vi "MultisitePinMapARegistered_SessionManagementApiRoundTrip_AllNodesSucceed.vi"() -> (6 "pass":bool, 8 "result":string, 15 "error out":errorcluster)   [LabVIEW 2020]
uses:
  Pin Map Client_lv/Pin Map Client_v1/RPC Messages/ni_measurementlink_pinmap_v1_CreatePinMapFromXmlRequest.ctl
  31aaf20a-e7c9-45c8-9685-a1adea383544.vi
  030eba9d-dfb1-4c70-a755-4ca582c4358b.vi
  <vilib>/Comparison/Less/Less Functor/Less Functor.lvclass
  Session Management Client_lv/Session Management Client_v1/Session Management Client_v1.lvlib
  Pin Map Client_lv/Pin Map Client_v1/Pin Map Client_v1.lvlib
panel:
  # "Test assumes discovery service, pin map service, and session management service have already been started."
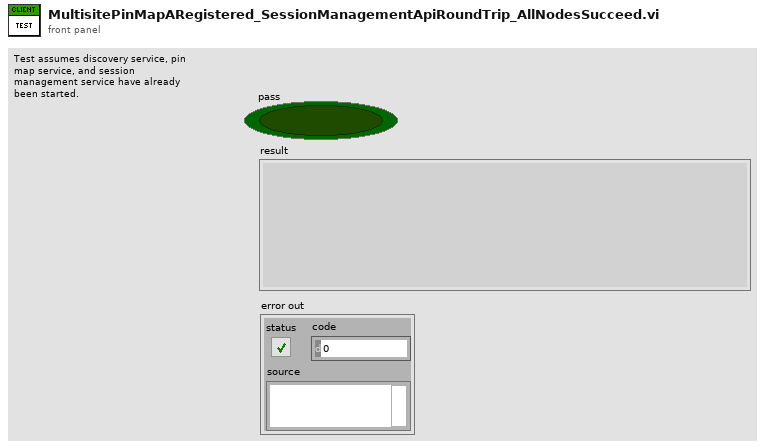
[diagram p1: front panel]
types:
  T1 = typedef "Pin Map Client_v1.lvlib/ni_measurementlink_pinmap_v1_CreatePinMapFromXmlRequest.ctl" = cluster{"pin_map_id":string, "pin_map_xml":string}
  T2 = typedef "grpc-lvsupport-release.lvlib/grpcId.ctl" = u64
  T3 = typedef "Session Management Client_v1.lvlib/ni_measurementlink_sessionmanagement_v1_ReserveSessionsRequest.ctl" = cluster{"pin_map_context":T4, "pin_or_relay_names":string[], "instrument_type_id":string, "timeout_in_milliseconds":i32}
  T4 = typedef "Session Management Client_v1.lvlib/ni_measurementlink_PinMapContext.ctl" = cluster{"pin_map_id":string, "sites":i32[]}
  T5 = cluster{"Registration Request Data":T3, "Expected instrument_type_id/session(s)":string[]}[]
  T6 = typedef "Session Management Client_v1.lvlib/ni_measurementlink_sessionmanagement_v1_ReserveSessionsResponse.ctl" = cluster{"sessions":T7[]}
  T7 = typedef "Session Management Client_v1.lvlib/ni_measurementlink_sessionmanagement_v1_SessionInformation.ctl" = cluster{"session":T8, "resource_name":string, "channel_list":string, "instrument_type_id":string, "session_exists":bool}
  T8 = typedef "Session Management Client_v1.lvlib/ni_measurementlink_sessionmanagement_v1_Session.ctl" = cluster{"name":string}
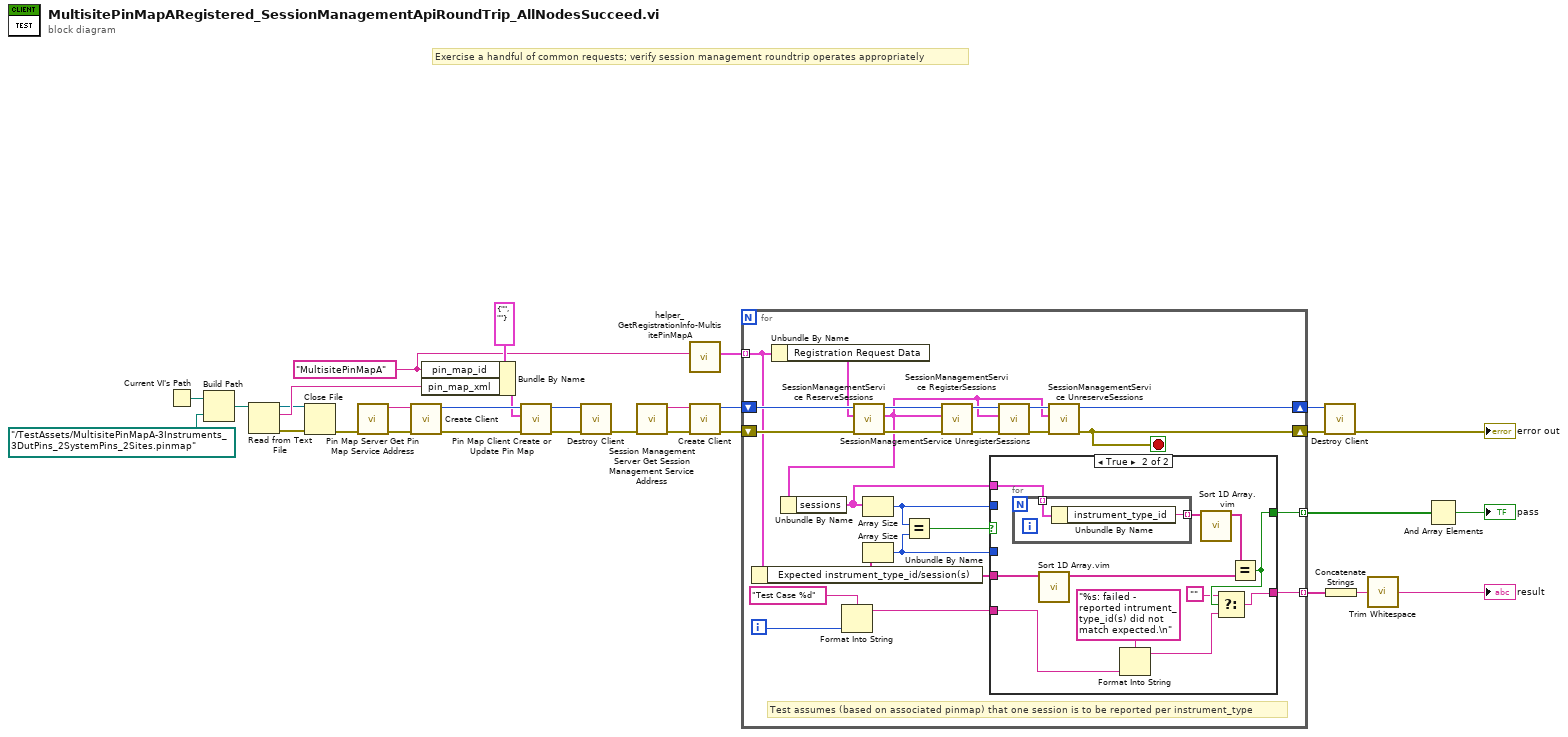
[diagram p0: block diagram]
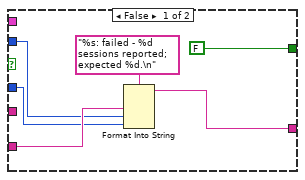
[diagram p2: hidden frame]
diagram:
  w7 = "MultisitePinMapA" ("pin_map_id")
  # "Exercise a handful of common requests; verify session management roundtrip operates appropriately"
  n1 = Current VI's Path() -> (path=w24:path)
  n2 = Build Path(base path=w24, name or relative path=path "../TestAssets/MultisitePinMapA-3Instruments_3DutPins_2SystemPins_2Sites.pinmap") -> (appended path=w22:path)
  n3 = Read from Text File(file (use dialog)=w22) -> (refnum out=w18:refnum<file>, text=w20:string, error out=w19:errorcluster)  [unwired: 3 in, 1 out]
  n4 = Close File(refnum=w18, error in=w19) -> (error out=w15:errorcluster)  [unwired: 1 out]
  n5 = call "Pin Map Server Get Pin Map Service Address.vi"("error in (no error)"=w15) -> ("error out"=w16:errorcluster, "address"=w17:string)  [unwired: 9 in]
  n6 = call "Create Client.vi"("error in"=w16, "address"=w17) -> ("error out"=w25:errorcluster, "gRPC ID Out"=w14:T2)  [unwired: 8 in]
  n7 = Bundle By Name(cluster=T1 {"pin_map_id"="", "pin_map_xml"=""} ("Request Data"), "pin_map_id"=w7, "pin_map_xml"=w20) -> (w13:T1)
  n8 = call "Pin Map Client Create or Update Pin Map.vi"("error in (no error)"=w25, "Request Data"=w13, "gRPC ID Out"=w14) -> ("error out"=w12:errorcluster, "gRPC ID out"=w11:T2)  [unwired: 6 in, 1 out]
  n9 = call "Destroy Client.vi"("error in"=w12, "gRPC ID"=w11) -> ("error out"=w10:errorcluster)  [unwired: 9 in]
  n10 = call "Session Management Server Get Session Management Service Address.vi"("error in (no error)"=w10) -> ("error out"=w29:errorcluster, "address"=w28:string)  [unwired: 9 in]
  n11 = call "helper_GetRegistrationInfo-MultisitePinMapA.vi"("Pin Map ID"=w7) -> ("Registration Request Info"=w6:T5)  [unwired: 10 in]
  n12 = call "Create Client.vi"("error in"=w29, "address"=w28) -> ("error out"=w27:errorcluster, "gRPC ID Out"=w26:T2)  [unwired: 8 in]
  n13 = for {
    shift-right: [w44] -> w8
    shift-left: w27 -> [w53]
    shift-right: [w46] -> w9
    shift-left: w26 -> [w52]
    tunnel: w6 -> [w36] mode=indexing
    tunnel: [w41] -> w5 mode=indexing
    tunnel: [w37] -> w3 mode=indexing
    i -> [w39]
    stop <- w44 stop-if-true
    # "Test assumes (based on associated pinmap) that one session is to be reported per instrument_type"
    n14 = Unbundle By Name(w36) -> ("Expected instrument_type_id/session(s)"=w31:string[])
    n15 = Unbundle By Name(w36) -> ("Registration Request Data"=w43:T3)
    n16 = Format Into String(format string="Test Case %d", w39) -> (resulting string=w38:string)  [unwired: 2 in, 1 out]
    n17 = call "SessionManagementService ReserveSessions.vi"("error in"=w53, "Request Data"=w43, "gRPC ID"=w52) -> ("error out"=w48:errorcluster, "Response Data"=w42:T6, "gRPC ID out"=w49:T2)  [unwired: 6 in]
    n18 = Unbundle By Name(w42) -> ("sessions"=w35:T7[])
    n19 = Array Size(array=w35) -> (size(s)=w33:i32)
    n20 = Array Size(array=w31) -> (size(s)=w32:i32)
    n21 = Equal?(x=w33, y=w32) -> (x = y?=w34:bool)
    n22 = call "SessionManagementService RegisterSessions.vi"("error in"=w48, "Request Data"=w42, "gRPC ID"=w49) -> ("error out"=w50:errorcluster, "gRPC ID out"=w51:T2)  [unwired: 6 in, 1 out]
    n23 = case shown="True" w34 {
      tunnel: [FALSE ("pass") w64] -> w41
      tunnel: w38 -> [w57 w60]
      tunnel: [w56 w65] -> w37
      tunnel: w35 -> [_ w70]
      tunnel: w33 -> [w55 _]
      tunnel: w32 -> [w54 _]
      tunnel: w31 -> [_ w68]
      frame False {
        n24 = Format Into String(format string="%s: failed - %d sessions reported; expected %d.\n", w57, w55, w54) -> (resulting string=w56:string)  [unwired: 2 in, 1 out]
      }
      frame True {
        n25 = for {
          tunnel: w70 -> [w72] mode=indexing
          tunnel: [w71] -> w69 mode=indexing
          n26 = Unbundle By Name(w72) -> ("instrument_type_id"=w71:string)
        }
        n27 = call "Sort 1D Array.vim"("unsorted array"=w68) -> ("sorted array"=w67:string[])  [unwired: 10 in]
        n28 = Format Into String(format string="%s: failed - reported intrument_type_id(s) did not match expected.\n", w60) -> (resulting string=w62:string)  [unwired: 2 in, 1 out]
        n29 = call "Sort 1D Array.vim"("unsorted array"=w69) -> ("sorted array"=w66:string[])  [unwired: 10 in]
        n30 = Equal?(x=w66, y=w67) -> (x = y?=w64:bool)
        n31 = Select(t="", s=w64, f=w62) -> (s? t:f=w65:string)
      }
    }
    n32 = call "SessionManagementService UnregisterSessions.vi"("error in"=w50, "Request Data"=w42, "gRPC ID"=w51) -> ("error out"=w45:errorcluster, "gRPC ID out"=w47:T2)  [unwired: 6 in, 1 out]
    n33 = call "SessionManagementService UnreserveSessions.vi"("error in"=w45, "Request Data"=w42, "gRPC ID"=w47) -> ("error out"=w44:errorcluster, "gRPC ID out"=w46:T2)  [unwired: 6 in, 1 out]
  }
  n34 = call "Destroy Client.vi"("error in"=w8, "gRPC ID"=w9) -> ("error out"=→"error out":errorcluster)  [unwired: 9 in]
  n35 = Concatenate Strings(w3) -> (w2:string)
  n36 = call <vilib>:"Trim Whitespace.vi"("string"=w2) -> ("trimmed string"=→"result":string)  [unwired: 1 in]
  n37 = And Array Elements(Boolean array=w5) -> (logical AND=→"pass":bool)
